vi "ParserPropertyPath.vi"(9 "Seleted Item Name":string="c") -> (2 "Property":string, 3 "Physical channel":string)   [LabVIEW 2017]
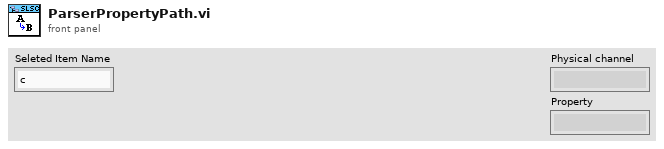
[diagram p1: front panel]
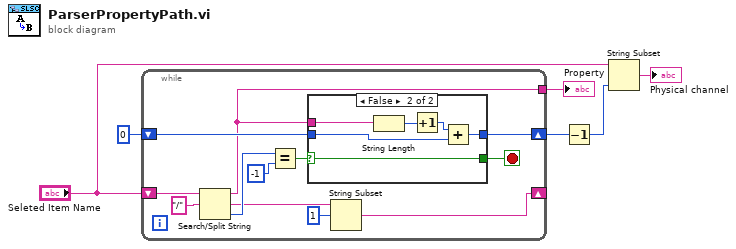
[diagram p0: block diagram]
diagram:
  n1 = while {
    shift-right: [w15] -> _
    shift-left: "Seleted Item Name" -> [w18]
    tunnel: [w7] -> w3
    shift-right: [w9] -> w5
    shift-left: 0 -> [w8]
    stop <- w10 stop-if-true
    n2 = Search/Split String(string=w18, search string/char (-)="/") -> (substring before match=w7:string, match + rest of string=w11:string, offset of match=w13:i32)  [unwired: 1 in]
    n3 = Equal?(x=w13, y=-1) -> (x = y?=w12:bool)
    n4 = case shown="False" w12 {
      selector: w12 -> [w20 w25]
      tunnel: w7 -> [_ w26]
      tunnel: [w20 w25] -> w10
      tunnel: [w19 w23] -> w9
      tunnel: w8 -> [w19 w21]
      frame True {
      }
      frame False {
        n5 = String Length(string=w26) -> (length=w24:i32)
        n6 = Increment(x=w24) -> (x+1=w22:i32)
        n7 = Add(x=w22, y=w21) -> (x+y=w23:i32)
      }
    }
    n8 = String Subset(string=w11, offset (0)=1) -> (substring=w15:string)  [unwired: 1 in]
  }
  "Property" <- w3
  n9 = Decrement(x=w5) -> (x-1=w2:i32)
  n10 = String Subset(string="Seleted Item Name", length (rest)=w2) -> (substring=→"Physical channel":string)  [unwired: 1 in]
